vi "OpAMP.vi"(1 "Max Amplitude":dbl, 2 "Analog Signal":waveform(dbl)) -> (0 "Amplified signal":waveform(dbl))   [LabVIEW 2013]
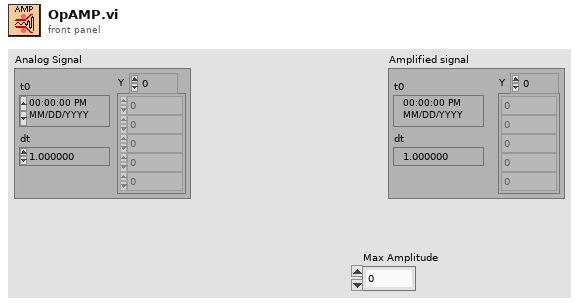
[diagram p1: front panel]
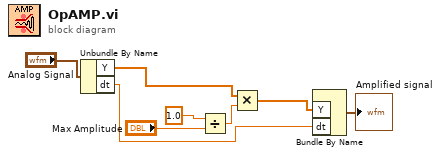
[diagram p0: block diagram]
diagram:
  n1 = Unbundle By Name("Analog Signal") -> ("Y"=w4:dbl[], "dt"=w2:dbl)
  n2 = Divide(x=1.0, y="Max Amplitude") -> (x/y=w6:dbl)
  n3 = Multiply(x=w4, y=w6) -> (x*y=w3:dbl[])
  n4 = Bundle By Name("Y"=w3, "dt"=w2) -> (→"Amplified signal":waveform(dbl))  [unwired: 1 in]
